vi "SENS_CORR_RPOW_OFFS_AMPL.vi"(0 "VISA IN":refnum<visa-resource-name>, 1 "Offset(dB)":i32, 5 "error in":errorcluster, 7 "Channel":i32) -> (14 "VISA Out":refnum<visa-resource-name>, 19 "error out":errorcluster)   [LabVIEW 2018, in "PNA-X.lvlib"]
doc: "SENSe<cnum>:CORRection:RPOWer:OFFSet[:AMPLitude] <num> \n(Read-Write) Adjusts a receiver power cal to account for components or adapters that are added \nbetween the source port and receiver while performing this cal. For more information, see Receiver \nCal. \nParameters \n<cnum> Any existing channel number. If unspecified, value is set to 1 \n<num> Offset Value in dB. Specify loss as a negative number; and gain as a positive \nnumber. Choose a number between -200 and 200. \nExamples SENS:CORR:RPOW:OFFS .5 \nsense2:correction:rpower:offset:amplitude .-5 \nQuery Syntax SENSe<cnum>:CORRection:RPOWer:OFFSet[:AMPLitude]? \nReturn Type Numeric \nDefault 0"
uses:
  PNA-X.lvlib
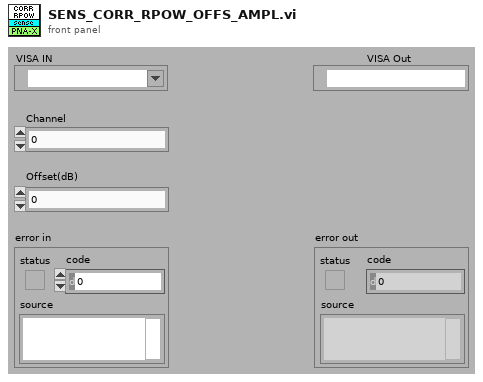
[diagram p1: front panel]
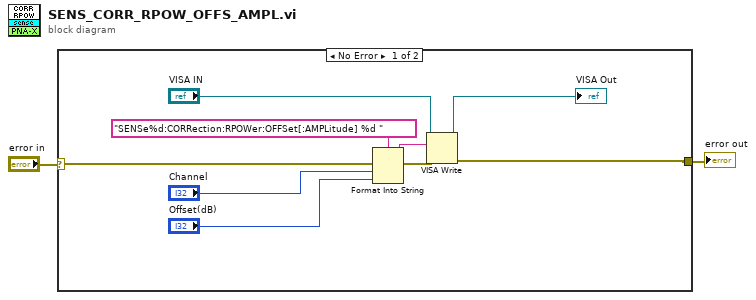
[diagram p0: block diagram]
diagram:
  n1 = case shown="No Error" "error in" {
    selector: "error in" -> [w11 w12]
    tunnel: [w6 w12] -> w1
    frame No Error {
      n2 = Format Into String(format string="SENSe%d:CORRection:RPOWer:OFFSet[:AMPLitude] %d " ("Cmdline"), error in=w11, "Channel", "Offset(dB)") -> (resulting string=w9:string, error out=w10:errorcluster)  [unwired: 1 in]
      n3 = VISA Write(VISA resource name="VISA IN", write buffer=w9, error in (no error)=w10) -> (VISA resource name out=→"VISA Out":refnum<visa-resource-name>, error out=w6:errorcluster)  [unwired: 1 out]
    }
    frame Error {
    }
  }
  "error out" <- w1
